vi "Binomial Coefficient.vi"(2 "k":u32, 3 "n":u32=1) -> (0 "error":i32, 1 "binomial coefficient (n,k)":dbl=1.0)   [LabVIEW 2010, in "NI_Gmath.lvlib"]
doc: "Calculates the binomial coefficient for nonnegative integer values of <B>n</B> and <B>k</B>."
uses:
  NI_Gmath.lvlib
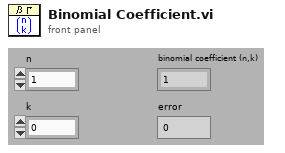
[diagram p1: front panel]
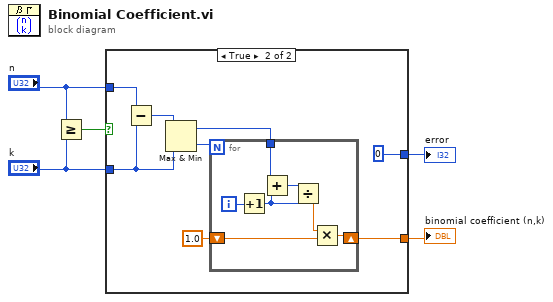
[diagram p0: block diagram]
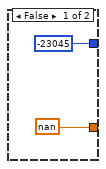
[diagram p2: hidden frame]
diagram:
  n1 = Greater Or Equal?(x="n", y="k") -> (x >= y?=w1:bool)
  n2 = case shown="True" w1 {
    tunnel: [nan w11] -> w5
    tunnel: [-23045 0] -> w4
    tunnel: "n" -> [_ w9]
    tunnel: "k" -> [_ w14]
    frame False {
    }
    frame True {
      n3 = Subtract(x=w9, y=w14) -> (x-y=w15:u32)
      n4 = Max & Min(x=w15, y=w14) -> (max(x,y)=w8:u32, min(x,y)=w13:u32)
      n5 = for {
        N: w13 -> [_]
        shift-right: [w17] -> w11
        shift-left: 1.0 -> [w19]
        tunnel: w8 -> [w22]
        i -> [w20]
        n6 = Increment(x=w20) -> (x+1=w16:i32)
        n7 = Add(x=w22, y=w16) -> (x+y=w21:u32)
        n8 = Divide(x=w21, y=w16) -> (x/y=w18:dbl)
        n9 = Multiply(x=w18, y=w19) -> (x*y=w17:dbl)
      }
    }
  }
  "binomial coefficient (n,k)" <- w5
  "error" <- w4
